vi "Configure Safe Power Down Sequence.vi"(0 "Instrument handle IN":refnum<k15>[](array[refnum]), 1 "Measurement Configuration":T2={"Quick Power Down"=FALSE, "Pin Name"=[], "Source Mode"=[], "Start Value"=[], "Target Value"=[], "Compliance Limit"=[], "Sense Mode"=[], "Default Ramp Rate"=[], "Ramp Rate"=[], "Start Delay"=[], "Relative To"=[], "Transient Response"=[], "Data Capture"=FALSE, "Power line frequency"=1} {"Relative To" items=["Power sequence start", "Previous source start", "Previous source end"]; "Power line frequency" items=["50 Hz", "60 Hz"]; "Start Value" format="%#_6p"; "Transient Response" items=["Slow", "Normal", "Fast"]; "Sense Mode" items=["Local Sense", "Remote Sense"]; "Target Value" format="%#_6p"; "Source Mode" items=["DC Voltage", "DC Current"]; "Start Delay" format="%#_6p"; "Compliance Limit" format="%#_6p"; "Ramp Rate" format="%#_6p"}, 5 "Channel Name":string[](array[string]), 7 "Ramp Configurations":T1, 11 "error in (no error)":errorcluster) -> (4 "Instrument Handle OUT":refnum<k15>[](array[refnum]), 6 "Advanced Sequence Created?":bool[](array[boolean]), 15 "error out":errorcluster)   [LabVIEW 2024, in "devicePowerSequencerCoreLogic.lvlib"]
uses:
  devicePowerSequencerCoreLogic.lvlib
  Measurement Configuration.ctl
  controls/Source Mode.ctl
  controls/Sense Mode.ctl
  controls/Relative To.ctl
  controls/Transient Response.ctl
  controls/Power line frequency.ctl
  controls/Ramp Configurations.ctl
  <instrlib>/niDCPower/nidcpower.llb/niDCPower Sequence Attribute Type.ctl
  <instrlib>/niDCPower/nidcpower.llb/niDCPower Create Advanced Sequence Commit Step With Channels.vi
  <instrlib>/niDCPower/nidcpower.llb/niDCPower Create Advanced Sequence Step With Channels.vi
  Device Power Sequencer.lvlib
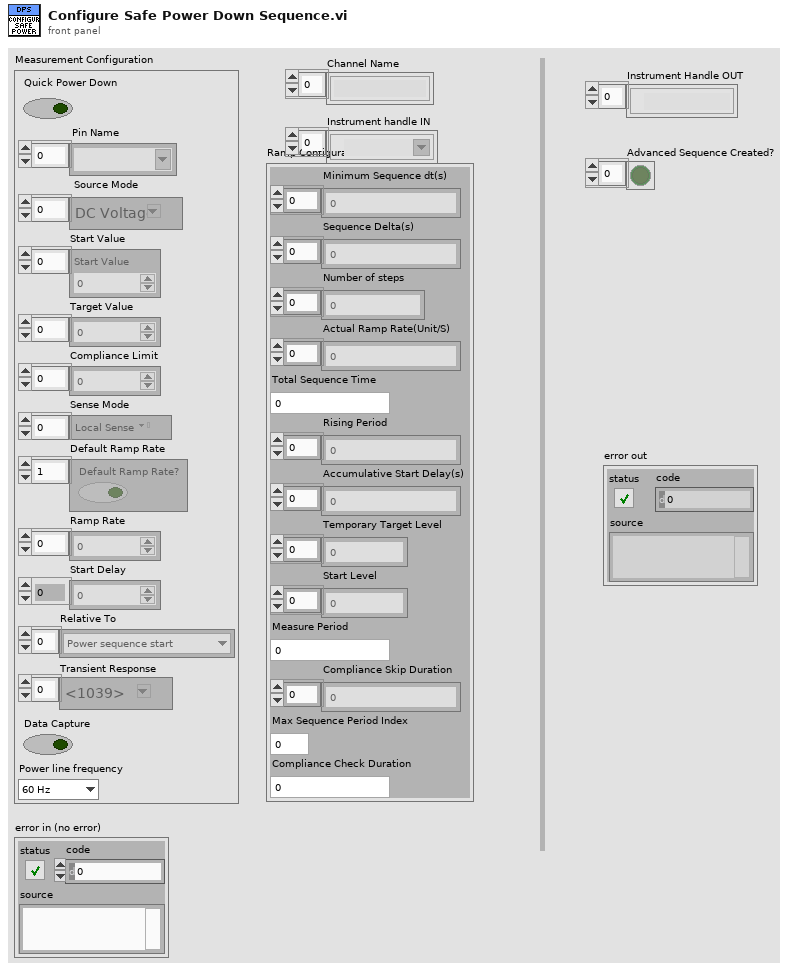
[diagram p1: front panel]
types:
  T1 = typedef "devicePowerSequencerCoreLogic.lvlib/Ramp Configurations.ctl" = cluster{"Minimum Sequence dt(s)":dbl[], "Sequence Delta(s)":dbl[], "Number of steps":i32[], "Actual Ramp Rate(Unit/S)":dbl[], "Total Sequence Time":dbl, "Rising Period":dbl[], "Accumulative Start Delay(s)":dbl[], "Temporary Target Level":dbl[], "Start Level":dbl[], "Measure Period":dbl, "Compliance Skip Duration":dbl[], "Max Sequence Period Index":i32, "Compliance Check Duration":dbl}
  T2 = typedef "Device Power Sequencer.lvlib/Measurement Configuration.ctl" = cluster{"Quick Power Down":bool, "Pin Name":string[], "Source Mode":T3[], "Start Value":dbl[], "Target Value":dbl[], "Compliance Limit":dbl[], "Sense Mode":T4[], "Default Ramp Rate":bool[], "Ramp Rate":dbl[], "Start Delay":dbl[], "Relative To":T5[], "Transient Response":T6[], "Data Capture":bool, "Power line frequency":T7}
  T3 = typedef "Device Power Sequencer.lvlib/Source Mode.ctl" = i32
  T4 = typedef "Device Power Sequencer.lvlib/Sense Mode.ctl" = i32
  T5 = typedef "Device Power Sequencer.lvlib/Relative To.ctl" = u32
  T6 = typedef "Device Power Sequencer.lvlib/Transient Response.ctl" = i32
  T7 = typedef "Device Power Sequencer.lvlib/Power line frequency.ctl" = u32
  T8 = typedef "niDCPower Sequence Attribute Type.ctl" = i32
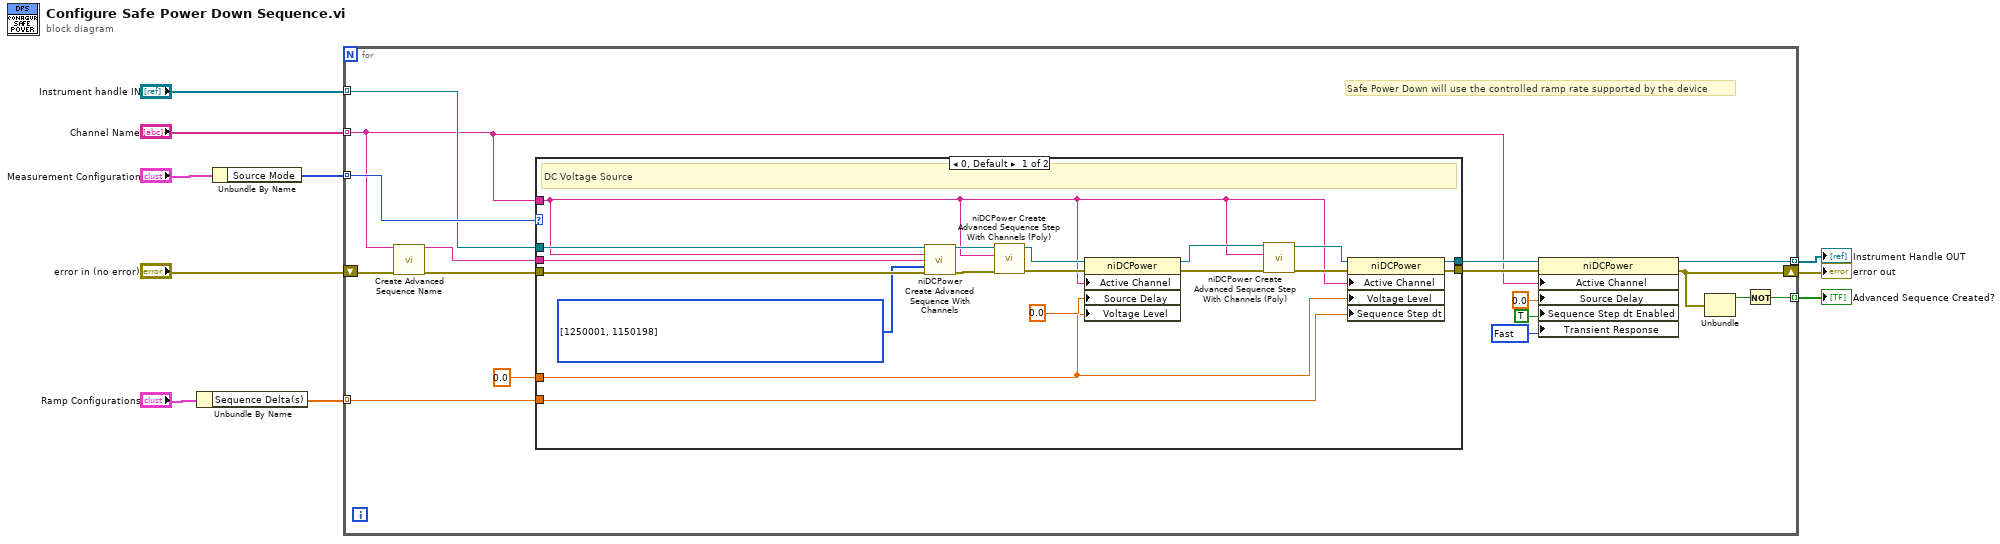
[diagram p0: block diagram]
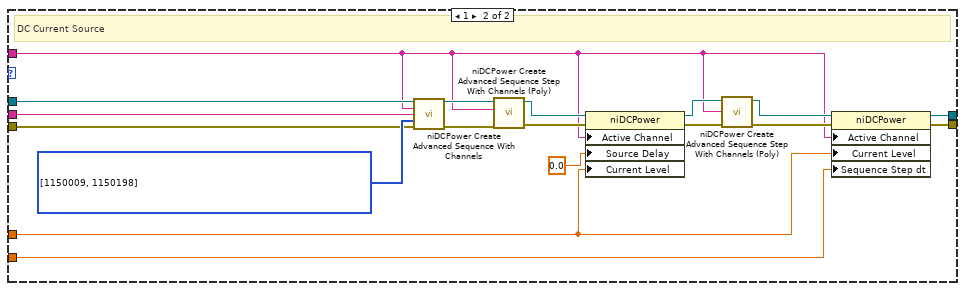
[diagram p2: hidden frame]
diagram:
  n1 = Unbundle By Name("Ramp Configurations") -> ("Sequence Delta(s)"=w7:dbl[])
  n2 = Unbundle By Name("Measurement Configuration") -> ("Source Mode"=w2:T3[])
  n3 = for {
    tunnel: "Instrument handle IN" -> [w19] mode=indexing
    tunnel: w7 -> [w16] mode=indexing
    tunnel: "Channel Name" -> [w11] mode=indexing
    shift-right: [w13] -> w4
    shift-left: "error in (no error)" -> [w18]
    tunnel: [w14] -> w3 mode=indexing
    tunnel: w2 -> [w22] mode=indexing
    tunnel: [w20] -> w1 mode=indexing
    w25 = 1039 items=["Slow"=1041, "Normal"=1038, "Fast"=1039, "Custom"=1042] ("Source:Transient Response")
    # "Safe Power Down will use the controlled ramp rate supported by the device"
    n4 = call "Create Advanced Sequence Name.vi"("Channel Name"=w11, "error in (no error)"=w18) -> ("String"=w12:string, "error out"=w17:errorcluster)  [unwired: 12 in]
    n5 = case shown="0, Default" w22 {
      tunnel: [w45 w63] -> w27
      tunnel: [w44 w62] -> w23
      tunnel: w19 -> [w37 w53]
      tunnel: w17 -> [w38 w55]
      tunnel: w16 -> [w43 w61]
      tunnel: w11 -> [w28 w46]
      tunnel: 0.0 -> [w29 w47]
      tunnel: w12 -> [w33 w52]
      frame 0, Default {
        w34 = T8[] [1250001, 1150198] items=["Source -> Output Function"=1150008, "Source -> Output Enabled"=1250006, "Source -> Output Resistance"=1150061, "Source -> Transient Response"=1150062, "Source -> Custom Transient Response -> Voltage Gain Bandwidth"=1150067, "Source -> Custom Transient Response -> Voltage Compensation Frequency"=1150068, "Source -> Custom Transient Response -> Voltage Pole-Zero Ratio"=1150069, "Source -> Custom Transient Response -> Current Gain Bandwidth"=1150070, "Source -> Custom Transient Response -> Current Compensation Frequency"=1150071, "Source -> Custom Transient Response -> Current Pole-Zero Ratio"=1150072, "Source -> DC Voltage -> Voltage Level"=1250001, "Source -> DC Voltage -> Voltage Level Range"=1150005, "Source -> DC Voltage -> Current Limit"=1250005, "Source -> DC Voltage -> Current Limit High"=1150187, "Source -> DC Voltage -> Current Limit Low"=1150188, "Source -> DC Voltage -> Current Limit Range"=1150004, "Source -> DC Current -> Current Level"=1150009, "Source -> DC Current -> Current Level Range"=1150011, "Source -> DC Current -> Voltage Limit"=1150010, "Source -> DC Current -> Voltage Limit High"=1150185, "Source -> DC Current -> Voltage Limit Low"=1150186, "Source -> DC Current -> Voltage Limit Range"=1150012, "Source -> Pulse Voltage -> Pulse Voltage Level"=1150080, "Source -> Pulse Voltage -> Pulse Bias Voltage Level"=1150082, "Source -> Pulse Voltage -> Pulse Voltage Level Range"=1150084, "Source -> Pulse Voltage -> Pulse Current Limit"=1150081, "Source -> Pulse Voltage -> Pulse Current Limit High"=1150193, "Source -> Pulse Voltage -> Pulse Current Limit Low"=1150194, "Source -> Pulse Voltage -> Pulse Bias Current Limit"=1150083, "Source -> Pulse Voltage -> Pulse Bias Current Limit High"=1150195, "Source -> Pulse Voltage -> Pulse Bias Current Limit Low"=1150196, "Source -> Pulse Voltage -> Pulse Current Limit Range"=1150085, "Source -> Pulse Current -> Pulse Current Level"=1150086, "Source -> Pulse Current -> Pulse Bias Current Level"=1150088, "Source -> Pulse Current -> Pulse Current Level Range"=1150090, "Source -> Pulse Current -> Pulse Voltage Limit"=1150087, "Source -> Pulse Current -> Pulse Voltage Limit High"=1150189, "Source -> Pulse Current -> Pulse Voltage Limit Low"=1150190, "Source -> Pulse Current -> Pulse Bias Voltage Limit"=1150089, "Source -> Pulse Current -> Pulse Bias Voltage Limit High"=1150191, "Source -> Pulse Current -> Pulse Bias Voltage Limit Low"=1150192, "Source -> Pulse Current -> Pulse Voltage Limit Range"=1150091, "Source -> Advanced -> Source Delay"=1150051, "Source -> Advanced -> Pulse Bias Delay"=1150092, "Source -> Advanced -> Pulse On Time"=1150093, "Source -> Advanced -> Pulse Off Time"=1150094, "Source -> Advanced -> OVP Enabled"=1250002, "Source -> Advanced -> OVP Limit"=1250003, "Source -> Advanced -> Compliance Limit Symmetry"=1150184, "Source -> Advanced -> Sequence Step Delta Time"=1150198, "Measurement -> Sense"=1150013, "Measurement -> Aperture Time"=1150058, "Measurement -> Measure Record Length"=1150063, "Measurement -> Advanced -> DC Noise Rejection"=1150066, "Measurement -> Autorange"=1150244, "Measurement -> Advanced -> Autorange Behavior"=1150245, "Measurement -> Advanced -> Autorange Aperture Time Mode"=1150246, "Measurement -> Advanced -> Autorange Minimum Aperture Time"=1150247, "Measurement -> Advanced -> Autorange Minimum Aperture Time Units"=1150248, "Measurement -> Advanced -> Autorange Minimum Current Range"=1150255, "Measurement -> Advanced -> Autorange Minimum Voltage Range"=1150256, "Measurement -> Advanced -> Autorange Threshold Mode"=1150257, "Measurement -> Advanced -> Autorange Maximum Delay After Range Change"=1150322, "LCR -> Instrument Mode"=1150208, "LCR -> Source Delay Mode"=1150315, "LCR -> Measurement Time"=1150218, "LCR -> Custom Measurement Time"=1150258, "LCR -> AC Stimulus -> Function"=1150209, "LCR -> AC Stimulus -> Frequency"=1150210, "LCR -> AC Stimulus -> Voltage Amplitude"=1150211, "LCR -> AC Stimulus -> Current Amplitude"=1150212, "LCR -> AC Stimulus -> Advanced -> Voltage Range"=1150265, "LCR -> AC Stimulus -> Advanced -> Current Range"=1150267, "LCR -> DC Bias -> Source"=1150213, "LCR -> DC Bias -> Voltage Level"=1150214, "LCR -> DC Bias -> Current Level"=1150215, "LCR -> DC Bias -> Advanced -> Voltage Range"=1150266, "LCR -> DC Bias -> Advanced -> Current Range"=1150274, "LCR -> Compensation -> Open -> Enabled"=1150220, "LCR -> Compensation -> Open -> Conductance"=1150261, "LCR -> Compensation -> Open -> Susceptance"=1150262, "LCR -> Compensation -> Short -> Enabled"=1150221, "LCR -> Compensation -> Short -> Resistance"=1150263, "LCR -> Compensation -> Short -> Reactance"=1150264, "LCR -> Compensation -> Load -> Enabled"=1150222, "LCR -> Compensation -> Load -> Measured Resistance"=1150268, "LCR -> Compensation -> Load -> Measured Reactance"=1150269, "LCR -> Compensation -> Load -> Actual Resistance"=1150270, "LCR -> Compensation -> Load -> Actual Reactance"=1150271, "LCR -> Impedance Range -> Impedance Range"=1150217, "LCR -> Impedance Range -> Impedance Autorange"=1150216, "LCR -> Impedance Range -> Advanced -> Impedance Range Source"=1150321, "LCR -> Impedance Range -> Advanced -> Load Resistance"=1150318, "LCR -> Impedance Range -> Advanced -> Load Inductance"=1150319, "LCR -> Impedance Range -> Advanced -> Load Capacitance"=1150320] ("advanced sequence properties")
        # "DC Voltage Source"
        n6 = call <instrlib>:"niDCPower Create Advanced Sequence With Channels.vi"("instrument handle"=w37, "channel name"=w28, "sequence name"=w33, "advanced sequence properties"=w34, "error in (no error)"=w38) -> ("instrument handle out"=w36:refnum<k15>, "error out"=w35:errorcluster)  [unwired: 9 in]
        n7 = call-poly <instrlib>:"niDCPower Create Advanced Sequence Step With Channels (Poly).vi"("error in (no error)"=w35, "channel name"=w28, "instrument handle"=w36) -> ("error out"=w42:errorcluster, "instrument handle out"=w41:refnum<k15>)  [unwired: 7 in]
        n8 = property class="niDCPower"(reference=w41, error in=w42, "Active Channel"=w28, "Source Delay"=0.0 ("Source:Advanced:Source Delay"), "Voltage Level"=w29) -> (reference out=w40:refnum<k15>, error out=w39:errorcluster)
        n9 = call-poly <instrlib>:"niDCPower Create Advanced Sequence Step With Channels (Poly).vi"("error in (no error)"=w39, "channel name"=w28, "instrument handle"=w40) -> ("error out"=w32:errorcluster, "instrument handle out"=w31:refnum<k15>)  [unwired: 7 in]
        n10 = property class="niDCPower"(reference=w31, error in=w32, "Active Channel"=w28, "Voltage Level"=w29, "Sequence Step dt"=w43) -> (reference out=w45:refnum<k15>, error out=w44:errorcluster)
      }
      frame 1 {
        w56 = T8[] [1150009, 1150198] items=["Source -> Output Function"=1150008, "Source -> Output Enabled"=1250006, "Source -> Output Resistance"=1150061, "Source -> Transient Response"=1150062, "Source -> Custom Transient Response -> Voltage Gain Bandwidth"=1150067, "Source -> Custom Transient Response -> Voltage Compensation Frequency"=1150068, "Source -> Custom Transient Response -> Voltage Pole-Zero Ratio"=1150069, "Source -> Custom Transient Response -> Current Gain Bandwidth"=1150070, "Source -> Custom Transient Response -> Current Compensation Frequency"=1150071, "Source -> Custom Transient Response -> Current Pole-Zero Ratio"=1150072, "Source -> DC Voltage -> Voltage Level"=1250001, "Source -> DC Voltage -> Voltage Level Range"=1150005, "Source -> DC Voltage -> Current Limit"=1250005, "Source -> DC Voltage -> Current Limit High"=1150187, "Source -> DC Voltage -> Current Limit Low"=1150188, "Source -> DC Voltage -> Current Limit Range"=1150004, "Source -> DC Current -> Current Level"=1150009, "Source -> DC Current -> Current Level Range"=1150011, "Source -> DC Current -> Voltage Limit"=1150010, "Source -> DC Current -> Voltage Limit High"=1150185, "Source -> DC Current -> Voltage Limit Low"=1150186, "Source -> DC Current -> Voltage Limit Range"=1150012, "Source -> Pulse Voltage -> Pulse Voltage Level"=1150080, "Source -> Pulse Voltage -> Pulse Bias Voltage Level"=1150082, "Source -> Pulse Voltage -> Pulse Voltage Level Range"=1150084, "Source -> Pulse Voltage -> Pulse Current Limit"=1150081, "Source -> Pulse Voltage -> Pulse Current Limit High"=1150193, "Source -> Pulse Voltage -> Pulse Current Limit Low"=1150194, "Source -> Pulse Voltage -> Pulse Bias Current Limit"=1150083, "Source -> Pulse Voltage -> Pulse Bias Current Limit High"=1150195, "Source -> Pulse Voltage -> Pulse Bias Current Limit Low"=1150196, "Source -> Pulse Voltage -> Pulse Current Limit Range"=1150085, "Source -> Pulse Current -> Pulse Current Level"=1150086, "Source -> Pulse Current -> Pulse Bias Current Level"=1150088, "Source -> Pulse Current -> Pulse Current Level Range"=1150090, "Source -> Pulse Current -> Pulse Voltage Limit"=1150087, "Source -> Pulse Current -> Pulse Voltage Limit High"=1150189, "Source -> Pulse Current -> Pulse Voltage Limit Low"=1150190, "Source -> Pulse Current -> Pulse Bias Voltage Limit"=1150089, "Source -> Pulse Current -> Pulse Bias Voltage Limit High"=1150191, "Source -> Pulse Current -> Pulse Bias Voltage Limit Low"=1150192, "Source -> Pulse Current -> Pulse Voltage Limit Range"=1150091, "Source -> Advanced -> Source Delay"=1150051, "Source -> Advanced -> Pulse Bias Delay"=1150092, "Source -> Advanced -> Pulse On Time"=1150093, "Source -> Advanced -> Pulse Off Time"=1150094, "Source -> Advanced -> OVP Enabled"=1250002, "Source -> Advanced -> OVP Limit"=1250003, "Source -> Advanced -> Compliance Limit Symmetry"=1150184, "Source -> Advanced -> Sequence Step Delta Time"=1150198, "Measurement -> Sense"=1150013, "Measurement -> Aperture Time"=1150058, "Measurement -> Measure Record Length"=1150063, "Measurement -> Advanced -> DC Noise Rejection"=1150066, "Measurement -> Autorange"=1150244, "Measurement -> Advanced -> Autorange Behavior"=1150245, "Measurement -> Advanced -> Autorange Aperture Time Mode"=1150246, "Measurement -> Advanced -> Autorange Minimum Aperture Time"=1150247, "Measurement -> Advanced -> Autorange Minimum Aperture Time Units"=1150248, "Measurement -> Advanced -> Autorange Minimum Current Range"=1150255, "Measurement -> Advanced -> Autorange Minimum Voltage Range"=1150256, "Measurement -> Advanced -> Autorange Threshold Mode"=1150257, "Measurement -> Advanced -> Autorange Maximum Delay After Range Change"=1150322, "LCR -> Instrument Mode"=1150208, "LCR -> Source Delay Mode"=1150315, "LCR -> Measurement Time"=1150218, "LCR -> Custom Measurement Time"=1150258, "LCR -> AC Stimulus -> Function"=1150209, "LCR -> AC Stimulus -> Frequency"=1150210, "LCR -> AC Stimulus -> Voltage Amplitude"=1150211, "LCR -> AC Stimulus -> Current Amplitude"=1150212, "LCR -> AC Stimulus -> Advanced -> Voltage Range"=1150265, "LCR -> AC Stimulus -> Advanced -> Current Range"=1150267, "LCR -> DC Bias -> Source"=1150213, "LCR -> DC Bias -> Voltage Level"=1150214, "LCR -> DC Bias -> Current Level"=1150215, "LCR -> DC Bias -> Advanced -> Voltage Range"=1150266, "LCR -> DC Bias -> Advanced -> Current Range"=1150274, "LCR -> Compensation -> Open -> Enabled"=1150220, "LCR -> Compensation -> Open -> Conductance"=1150261, "LCR -> Compensation -> Open -> Susceptance"=1150262, "LCR -> Compensation -> Short -> Enabled"=1150221, "LCR -> Compensation -> Short -> Resistance"=1150263, "LCR -> Compensation -> Short -> Reactance"=1150264, "LCR -> Compensation -> Load -> Enabled"=1150222, "LCR -> Compensation -> Load -> Measured Resistance"=1150268, "LCR -> Compensation -> Load -> Measured Reactance"=1150269, "LCR -> Compensation -> Load -> Actual Resistance"=1150270, "LCR -> Compensation -> Load -> Actual Reactance"=1150271, "LCR -> Impedance Range -> Impedance Range"=1150217, "LCR -> Impedance Range -> Impedance Autorange"=1150216, "LCR -> Impedance Range -> Advanced -> Impedance Range Source"=1150321, "LCR -> Impedance Range -> Advanced -> Load Resistance"=1150318, "LCR -> Impedance Range -> Advanced -> Load Inductance"=1150319, "LCR -> Impedance Range -> Advanced -> Load Capacitance"=1150320] ("advanced sequence properties")
        # "DC Current Source"
        n11 = call <instrlib>:"niDCPower Create Advanced Sequence With Channels.vi"("instrument handle"=w53, "channel name"=w46, "sequence name"=w52, "advanced sequence properties"=w56, "error in (no error)"=w55) -> ("instrument handle out"=w51:refnum<k15>, "error out"=w54:errorcluster)  [unwired: 9 in]
        n12 = call-poly <instrlib>:"niDCPower Create Advanced Sequence Step With Channels (Poly).vi"("error in (no error)"=w54, "channel name"=w46, "instrument handle"=w51) -> ("error out"=w60:errorcluster, "instrument handle out"=w59:refnum<k15>)  [unwired: 7 in]
        n13 = property class="niDCPower"(reference=w59, error in=w60, "Active Channel"=w46, "Source Delay"=0.0 ("Source:Advanced:Source Delay"), "Current Level"=w47) -> (reference out=w58:refnum<k15>, error out=w57:errorcluster)
        n14 = call-poly <instrlib>:"niDCPower Create Advanced Sequence Step With Channels (Poly).vi"("error in (no error)"=w57, "channel name"=w46, "instrument handle"=w58) -> ("error out"=w50:errorcluster, "instrument handle out"=w49:refnum<k15>)  [unwired: 7 in]
        n15 = property class="niDCPower"(reference=w49, error in=w50, "Active Channel"=w46, "Current Level"=w47, "Sequence Step dt"=w61) -> (reference out=w63:refnum<k15>, error out=w62:errorcluster)
      }
    }
    n16 = property class="niDCPower"(reference=w27, error in=w23, "Active Channel"=w11, "Source Delay"=0.0 ("Source:Advanced:Source Delay"), "Sequence Step dt Enabled"=TRUE ("Source:Advanced:Sequence Step Delta Time Enabled"), "Transient Response"=w25) -> (reference out=w14:refnum<k15>, error out=w13:errorcluster)
    n17 = Unbundle(w13) -> ("status"=w21:bool)  [unwired: 2 out]
    n18 = Not(x=w21) -> (.not. x?=w20:bool)
  }
  "error out" <- w4
  "Instrument Handle OUT" <- w3
  "Advanced Sequence Created?" <- w1
